vi "InitCalibrationVolumes.vi"   [LabVIEW 2013]
uses:
  GlobalVariables/SystemParameters.vi
  GlobalVariables/CalibrationVolumes.vi
types:
  T1 = cluster{"defaultLanguage":string, "languageFile":string, "languages":string, "calibrationVolumeFile":string}
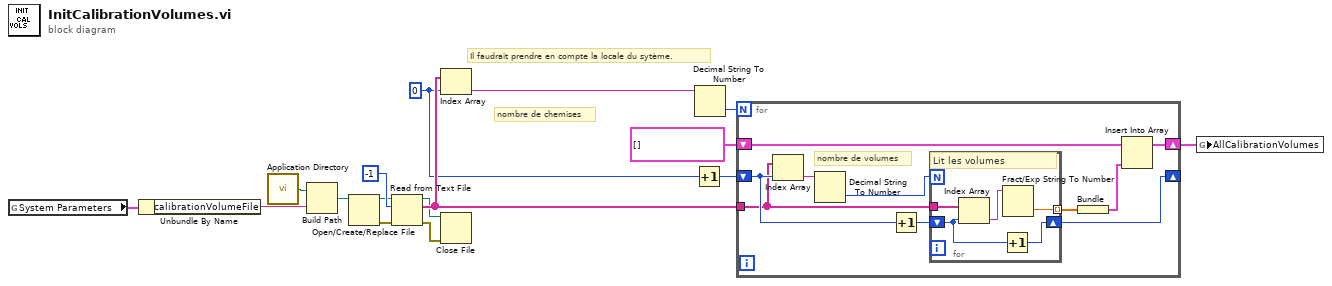
[diagram p0: block diagram]
diagram:
  w4 = 0
  # "Il faudrait prendre en compte la locale du sytème."
  # "nombre de chemises"
  n1 = global read "SystemParameters.vi" "System Parameters"() -> (w2:T1)
  n2 = Unbundle By Name(w2) -> ("calibrationVolumeFile"=w1:string)
  n3 = call <vilib>:"Application Directory.vi"() -> ("Application Directory"=w16:path)
  n4 = Build Path(base path=w16, name or relative path=w1) -> (appended path=w14:path)
  n5 = Open/Create/Replace File(file path (use dialog)=w14) -> (refnum out=w12:refnum<file>, error out=w13:errorcluster)  [unwired: 5 in, 1 out]
  n6 = Read from Text File(file (use dialog)=w12, count=-1, error in=w13) -> (refnum out=w7:refnum<file>, text=w8:string[], error out=w6:errorcluster)  [unwired: 1 in, 1 out]
  n7 = Index Array(array=w8, index=w4) -> (element=w9:string)
  n8 = Close File(refnum=w7, error in=w6) -> ()  [unwired: 2 out]
  n9 = Increment(x=w4) -> (x+1=w5:i32)
  n10 = Decimal String To Number(string=w9) -> (number=w3:i32)  [unwired: 2 in, 1 out]
  n11 = for {
    N: w3 -> [_]
    shift-right: [w23] -> w10
    shift-left: cluster{"CalibrationVolumes":dbl[]}[] [] ("AllCalibrationVolumes") -> [w24]
    shift-right: [w17] -> _
    shift-left: w5 -> [w20]
    tunnel: w8 -> [w18]
    # "nombre de volumes"
    n12 = Index Array(array=w18, index=w20) -> (element=w19:string)
    n13 = Decimal String To Number(string=w19) -> (number=w22:i32)  [unwired: 2 in, 1 out]
    n14 = Increment(x=w20) -> (x+1=w21:i32)
    n15 = for {
      N: w22 -> [_]
      tunnel: [w27] -> w26 mode=indexing
      shift-right: [w29] -> w17
      shift-left: w21 -> [w28]
      tunnel: w18 -> [w30]
      # "Lit les volumes"
      n16 = Index Array(array=w30, index=w28) -> (element=w31:string)
      n17 = Increment(x=w28) -> (x+1=w29:i32)
      n18 = Fract/Exp String To Number(string=w31) -> (number=w27:dbl)  [unwired: 3 in, 1 out]
    }
    n19 = Bundle(w26) -> (w25:cluster{dbl[]})  [unwired: 1 in]
    n20 = Insert Into Array(array=w24, new element=w25) -> (w23:cluster{"CalibrationVolumes":dbl[]}[])  [unwired: 1 in]
  }
  n21 = global write "CalibrationVolumes.vi" "AllCalibrationVolumes"(w10) -> ()
